vi "AxisConfiguration_Write.vi"(1 "AxisConfigurationIN":T1={"AxisHomeType"=1, "AxisBacklash"=0.0, "AxisGain"=1.0, "AxisOffset"=0.0, "AxisUnit"=0, "ReqConfRead"=FALSE, "ReqConfWrite"=FALSE, "AxisName"="", "AxisAccDecc"=0.0, "AxisHomeVel"=0.0} {"AxisUnit" items=["mm", "°"]; "AxisHomeType" items=["no homing"=0, "forward limit switch"=1, "backward limit switch"=2, "forward reference"=4, "backward reference"=8]}, 2 "AxisNo":u16) -> ()   [LabVIEW 2020, in "SMCD14_lib.lvlib"]
uses:
  SMCD14_lib.lvlib
  AxisConfiguration_typedef.ctl
  Globals.vi
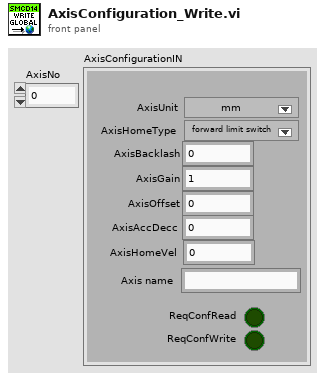
[diagram p1: front panel]
types:
  T1 = typedef "SMCD14_lib.lvlib/AxisConfiguration_typedef.ctl" = cluster{"AxisHomeType":u16, "AxisBacklash":dbl, "AxisGain":dbl, "AxisOffset":dbl, "AxisUnit":u16, "ReqConfRead":bool, "ReqConfWrite":bool, "AxisName":string, "AxisAccDecc":dbl, "AxisHomeVel":dbl}
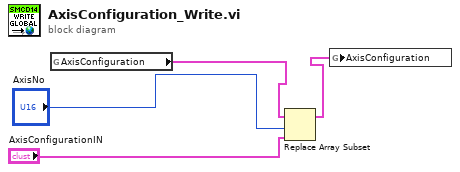
[diagram p0: block diagram]
diagram:
  n1 = global read "Globals.vi" "AxisConfiguration"() -> (w4:T1[])
  n2 = Replace Array Subset(array=w4, new element="AxisConfigurationIN", index="AxisNo") -> (w3:T1[])
  n3 = global write "Globals.vi" "AxisConfiguration"(w3) -> ()
